vi "getNearest.vi"(3 "error in (no error)":errorcluster, 4 "value":dbl, 5 "array":dbl[][](array[numeric])) -> (0 "error out":errorcluster, 1 "nearest value":dbl, 2 "nearest index":dbl)   [LabVIEW 2014, in "Array.lvlib"]
doc: "Use this template to build a VI to use as a subVI."
uses:
  Array.lvlib
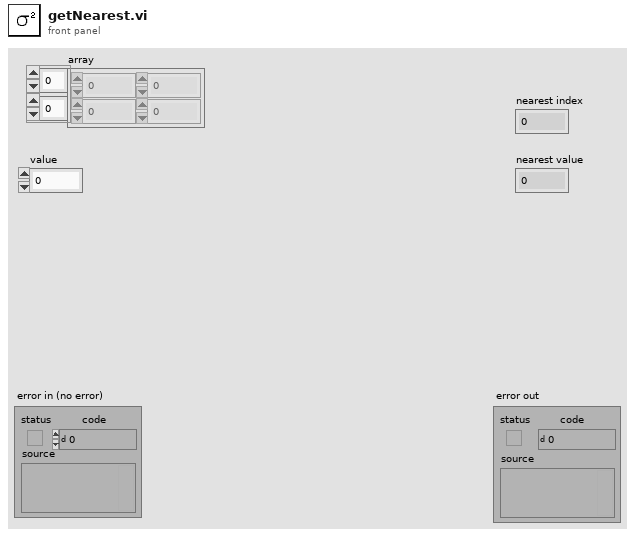
[diagram p1: front panel]
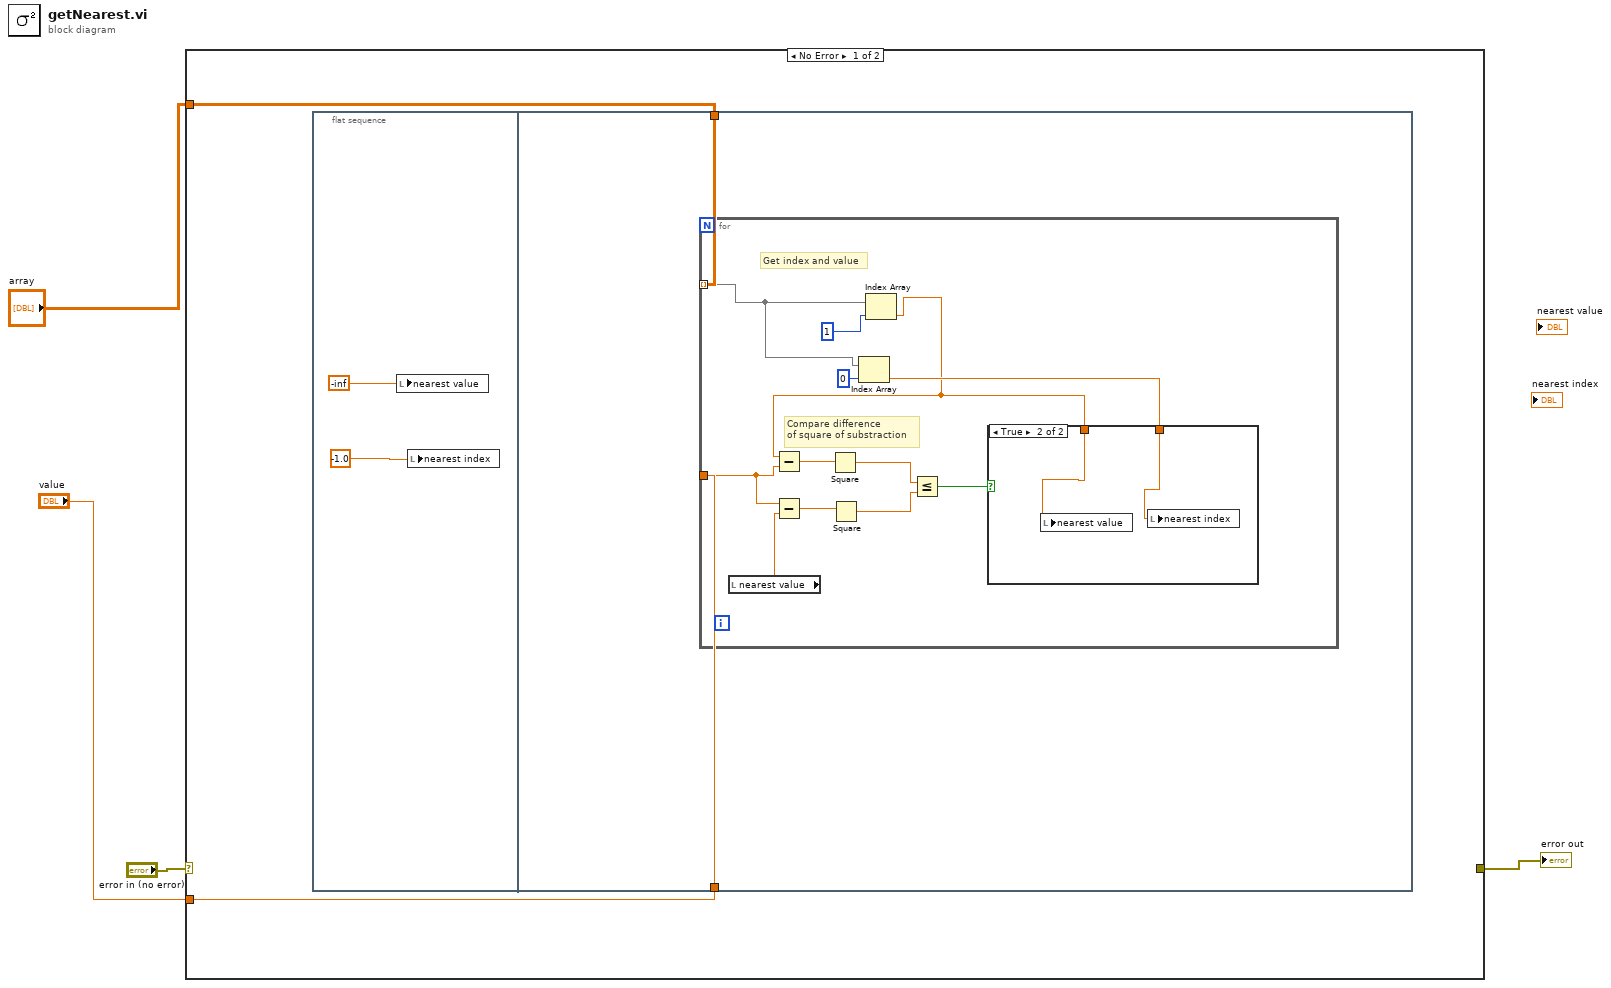
[diagram p0: block diagram]
diagram:
  n1 = case shown="No Error" "error in (no error)" {
    selector: "error in (no error)" -> [_ w25]
    tunnel: [_ w25] -> w3
    tunnel: "array" -> [w6 _]
    tunnel: "value" -> [w5 _]
    frame No Error {
      n2 = flat-sequence {
        tunnel: w6 -> [w10]
        tunnel: w5 -> [w9]
        frame #0 {
          n3 = local write "nearest value"(-inf) -> ()
          n4 = local write "nearest index"(-1.0 ("nearest index")) -> ()
        }
        frame #1 {
          n5 = for {
            tunnel: w10 -> [w14] mode=indexing
            tunnel: w9 -> [w17]
            # "Compare difference\nof square of substraction"
            # "Get index and value"
            n6 = local read "nearest value"() -> (w11:dbl)
            n7 = Subtract(x=w17, y=w11) -> (x-y=w19:dbl)
            n8 = Square(x=w19) -> (x^2=w18:dbl)
            n9 = Index Array(array=w14, index=0) -> (element=w13:dbl)
            n10 = Index Array(array=w14, index=1 ("index (dim 6)")) -> (element=w12:dbl)
            n11 = Subtract(x=w12, y=w17) -> (x-y=w21:dbl)
            n12 = Square(x=w21) -> (x^2=w20:dbl)
            n13 = Less Or Equal?(x=w20, y=w18) -> (x <= y?=w16:bool)
            n14 = case shown="True" w16 {
              tunnel: w13 -> [_ w24]
              tunnel: w12 -> [_ w23]
              frame False {
              }
              frame True {
                n15 = local write "nearest value"(w23) -> ()
                n16 = local write "nearest index"(w24) -> ()
              }
            }
          }
        }
      }
    }
    frame Error {
    }
  }
  "error out" <- w3
